vi "GetControlTermIdx.vi"(11 "ArrayElementScripter in":refnum<class "ArrayElementScripter.lvclass">) -> (2 "TermIdx":u32=2, 3 "ArrayElementScripter out":refnum<class "ArrayElementScripter.lvclass">)   [LabVIEW 2021, in "MemberVICreation.lvlib" / "ArrayElementScripter.lvclass"]
uses:
  <resource>/Framework/Providers/LVClassLibrary/NewAccessors/ArrayElementScripter/ArrayElementScripter.lvclass
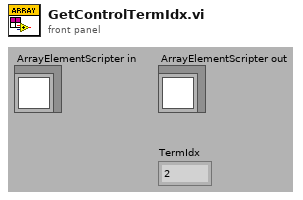
[diagram p1: front panel]
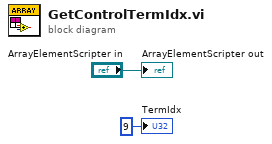
[diagram p0: block diagram]
diagram:
  "TermIdx" <- u32 9 ("TermIdx")
  "ArrayElementScripter out" <- "ArrayElementScripter in"
